vi "ReadChannels.vi"(7 "DigNum Refnum":refnum<vi>, 8 "error in (no error)":errorcluster, 9 "Task Name":string="Acquisition", 10 "MCListbox Refnum":refnum<vi>, 11 "Array in":refnum<vi>) -> (0 "error out":errorcluster)   [LabVIEW 2017, in "DAQConfig.lvlib"]
uses:
  DAQConfig.lvlib
  <resource>/objmgr/daqmx.rc
panel:
  out "ChanType":i32(ring)=10100 items=["Analog Input"=10100, "Analog Output"=10102, "Digital Input"=10151, "Digital Output"=10153, "Counter Input"=10131, "Counter Output"=10132]
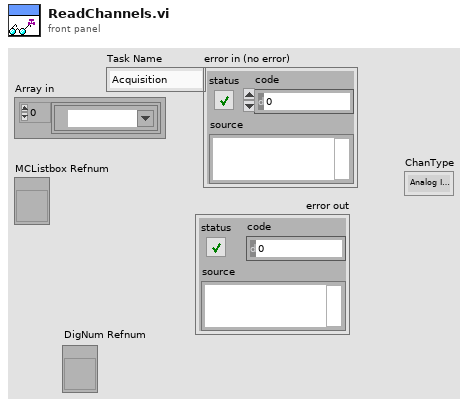
[diagram p1: front panel]
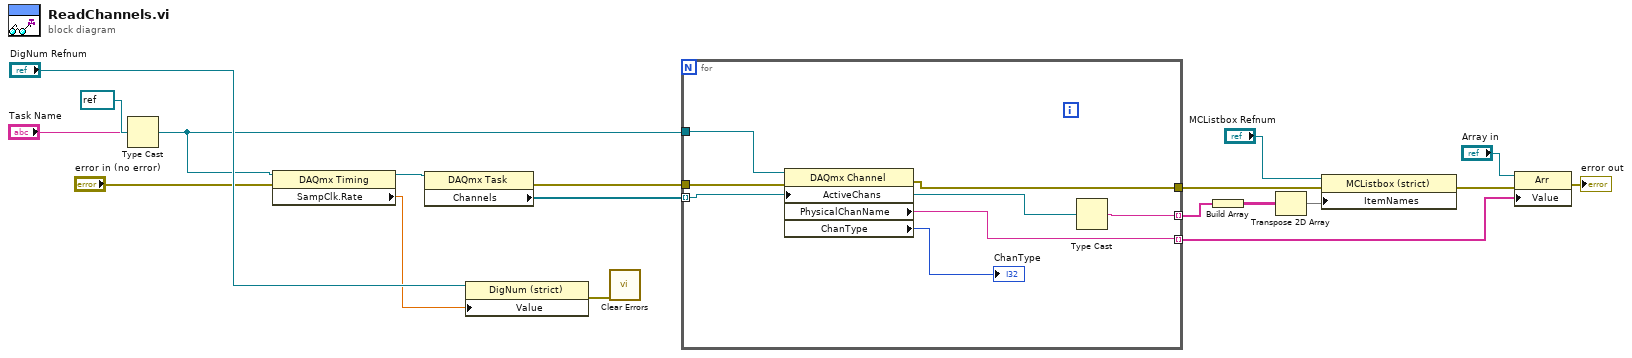
[diagram p0: block diagram]
diagram:
  n1 = Type Cast(type=refnum<k21> refnum ("task"), x="Task Name") -> (*(type *) &x=w5:refnum<k21>)
  n2 = property class="DAQmx Timing"(reference=w5, error in="error in (no error)") -> (reference out=w4:refnum<k21>, "SampClk.Rate"=w2:dbl)  [unwired: 1 out]
  n3 = property class="DAQmx Task"(reference=w4) -> (error out=w15:errorcluster, "Channels"=w17:refnum<k21>[])  [unwired: 1 in, 1 out]
  n4 = property class="DigNum (strict)"(reference="DigNum Refnum", "Value"=w2) -> (error out=w1:errorcluster)  [unwired: 1 in, 1 out]
  n5 = call <vilib>:"Clear Errors.vi"("error in (no error)"=w1) -> ()  [unwired: 5 in, 2 out]
  n6 = for {
    tunnel: w17 -> [w23] mode=indexing
    tunnel: w15 -> [w26]
    tunnel: w5 -> [w20]
    tunnel: [w25] -> w13 mode=indexing
    tunnel: [w22] -> w12 mode=indexing
    tunnel: [w21] -> w11
    n7 = property class="DAQmx Channel"(reference=w20, error in=w26, "ActiveChans"=w23) -> (error out=w21:errorcluster, "PhysicalChanName"=w25:tag, "ChanType"=→"ChanType":i32)  [unwired: 1 out]
    n8 = Type Cast(x=w23) -> (*(type *) &x=w22:string)  [unwired: 1 in]
  }
  n9 = Build Array(w12) -> (w8:string[][])
  n10 = Transpose 2D Array(2D array=w8) -> (transposed array=w7:string[][])
  n11 = property on="Property Node" class="MCListbox (strict)"(reference="MCListbox Refnum", error in=w11, "ItemNames"=w7) -> (error out=w10:errorcluster)  [unwired: 1 out]
  n12 = property class="Arr"(reference="Array in", error in=w10, "Value"=w13) -> (error out=→"error out":errorcluster)  [unwired: 1 out]
